vi "CRYWrite Recnet.vi"   [LabVIEW 2013]
doc: "Config File Reading/Writting\n\nPath \n ini File path\nRWFlag\n 0: no action\n 1: read\n 2: write"
uses:
  CRYMainGlobal.vi
panel:
  # "Save recent configuration."
types:
  T1 = cluster{"Section":string, "Item":cluster{"Key":string, "Value":string}[]}
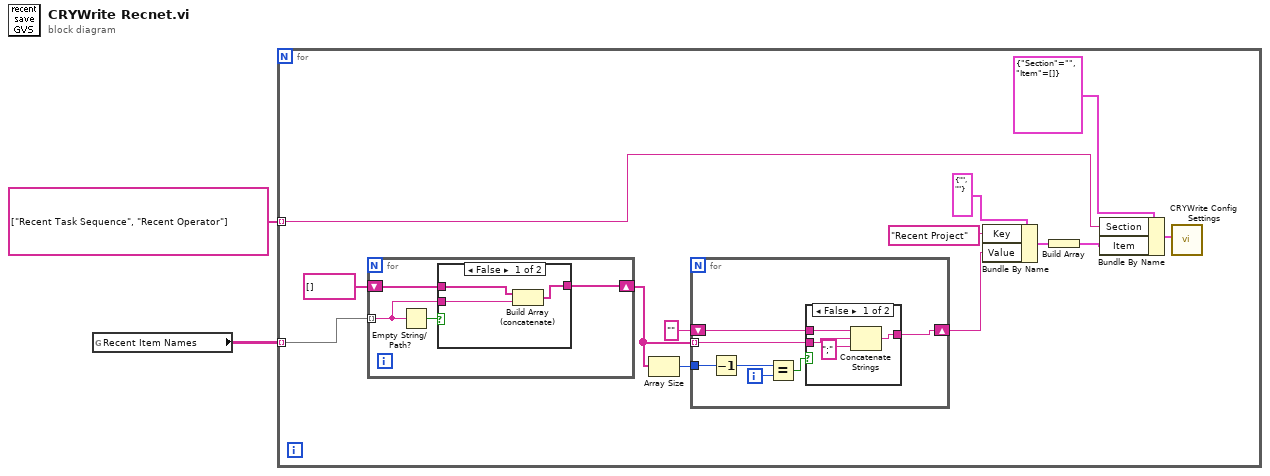
[diagram p0: block diagram]
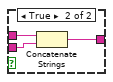
[diagram p3: hidden frame]
diagram:
  n1 = global read "CRYMainGlobal.vi" "Recent Item Names"() -> (w2:string[][])
  n2 = for {
    tunnel: w2 -> [w5] mode=indexing
    tunnel: string[] ["Recent Task Sequence", "Recent Operator"] -> [w6] mode=indexing
    n3 = for {
      tunnel: w5 -> [w18] mode=indexing
      shift-right: [w16] -> w3
      shift-left: string[] [] -> [w17]
      n4 = Empty String/Path?(string/path=w18) -> (empty?=w19:bool)
      n5 = case shown="False" w19 {
        tunnel: w18 -> [w22 _]
        tunnel: w17 -> [w21 w23]
        tunnel: [w20 w23] -> w16
        frame False {
          n6 = Build Array (concatenate)(w21, w22) -> (w20:string[])
        }
        frame True {
        }
      }
    }
    n7 = Array Size(array=w3) -> (size(s)=w15:i32)
    n8 = for {
      tunnel: w3 -> [w30] mode=indexing
      shift-right: [w29] -> w10
      shift-left: "" -> [w28]
      tunnel: w15 -> [w26]
      i -> [w27]
      n9 = Decrement(x=w26) -> (x-1=w25:i32)
      n10 = Equal?(x=w25, y=w27) -> (x = y?=w24:bool)
      n11 = case shown="False" w24 {
        tunnel: w30 -> [w34 w36]
        tunnel: [w33 w35] -> w29
        tunnel: w28 -> [w32 w37]
        frame False {
          n12 = Concatenate Strings(w32, w34, ";" ("string")) -> (w33:string)
        }
        frame True {
          n13 = Concatenate Strings(w37, w36) -> (w35:string)
        }
      }
    }
    n14 = Bundle By Name(cluster=cluster{"Key":string, "Value":string} {"Key"="", "Value"=""} ("Cluster"), "Key"="Recent Project" ("Section"), "Value"=w10) -> (w9:cluster{"Key":string, "Value":string})
    n15 = Build Array(w9) -> (w8:cluster{"Key":string, "Value":string}[])
    n16 = Bundle By Name(cluster=T1 {"Section"="", "Item"=[]}, "Section"=w6, "Item"=w8) -> (w7:T1)
    n17 = call "CRYWrite Config Settings.vi"("Config Data"=w7) -> ()  [unwired: 1 in, 8 out]
  }
